vi "Read_Map.vi"(8 "error_in":errorcluster, 11 "Image In":T1) -> (0 "error out":errorcluster)   [LabVIEW 2020]
uses:
  <vilib>/vision/Image Controls.llb/IMAQ Image.ctl
  <vilib>/vision/NI_Vision_Development_Module.lvlib
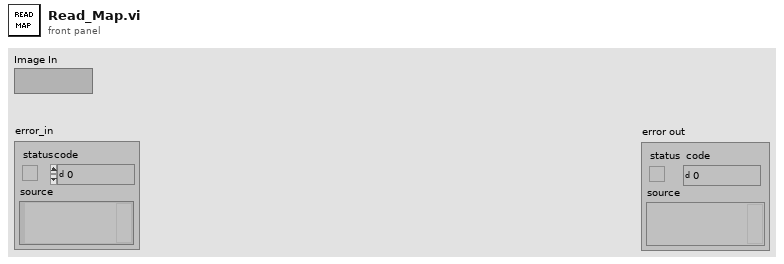
[diagram p1: front panel]
types:
  T1 = typedef "IMAQ Image.ctl" = refnum<image>
  T2 = typedef "Image_Cluster.ctl" = cluster{"Detector_info":cluster{"No. of detectors":dbl, "Detector_Array":string[][], "Detector_Array_Numeric":dbl[][]}, "Corner_info":cluster{"Corner_Array":dbl[][]}, "ROI":cluster{"Corners":cluster{"Global Rectangle":i32[], "Contours":cluster{"ID":enum32{"External", "Internal"}, "Type":u32, "Coordinates":i32[]}[]}[], "Detectors":cluster{"Global Rectangle":i32[], "Contours":cluster{"ID":enum32{"External", "Internal"}, "Type":u32, "Coordinates":i32[]}[]}[]}, "Shape_Detect":cluster{"Match_score":dbl, "Curve Parameters":T3, "Match Options":T4, "Circle Descriptor":cluster{"Min Radius":dbl, "Max Radius":dbl}}, "Path":cluster{"Config":path, "Map":path}, "Map":cluster{"X_resolution":i32, "Y_resolution":i32, "Image":T1}, "Conversion_factor":dbl}
  T3 = typedef "IMAQ Curve Parameters.ctl" = cluster{"Extraction Mode":u32, "Edge Threshold":i32, "Edge Filter Size":u32, "Min Length":i32, "Row Search Step Size":i32, "Col Search Step Size":i32, "Max Endpoint Gap":i32, "Closed":bool, "Subpixel":bool}
  T4 = typedef "ShapeDetectionMatchOptions.ctl" = cluster{"Rotation":bool, "Scale":bool, "Occlusion":bool, "Range Settings":T5[]}
  T5 = typedef "IMAQ Match Range Setting.ctl" = cluster{"Match Constraints":u32, "Min":dbl, "Max":dbl}
  T6 = cluster{"Global Rectangle":i32[], "Contours":cluster{"ID":enum32{"External", "Internal"}, "Type":u32, "Coordinates":i32[]}[]}[]
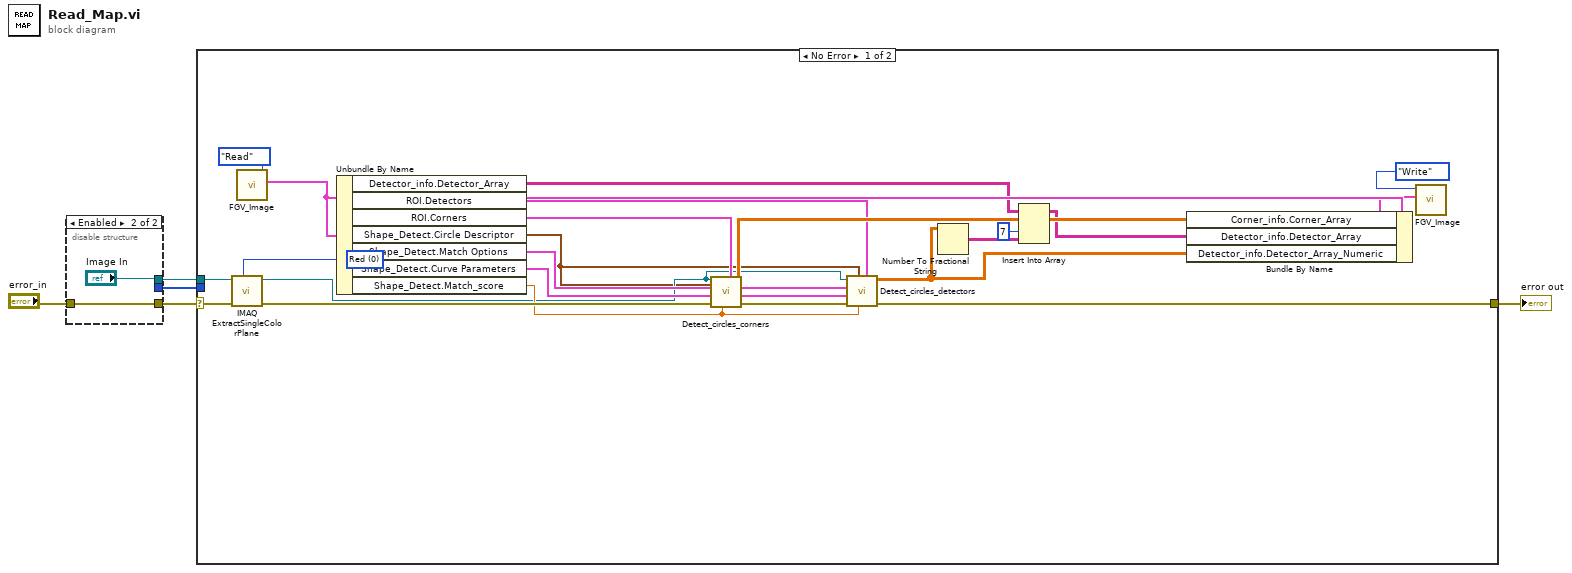
[diagram p0: block diagram]
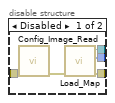
[diagram p2: hidden frame]
diagram:
  n1 = disable-structure shown="Enabled" {
    disable-tunnel: [w10 w12] -> w5
    disable-tunnel: [w9 "Image In"] -> w4
    disable-tunnel: [w8 _] -> w3
    disable-tunnel: "error_in" -> [w7 w12]
    frame Disabled {
      n2 = call "Config_Image_Read.vi"("error in (no error)"=w7) -> ("error out"=w6:errorcluster)  [unwired: 10 in]
      n3 = call "Load_Map.vi"("error in (no error)"=w6) -> ("error out"=w10:errorcluster, "image size"=w8:i32[], "Image Out"=w9:T1)  [unwired: 7 in]
    }
    frame Enabled {
    }
  }
  n4 = case shown="No Error" w5 {
    selector: w5 -> [w34 w36]
    tunnel: w4 -> [w35 _]
    tunnel: w3 -> [_ _]
    tunnel: [w24 w36] -> w2
    frame No Error {
      w26 = 0 items=["Red", "Green", "Blue", "Hue", "Saturation", "Luminance", "Value", "Intensity"] ("Color Plane")
      n5 = call "IMAQ ExtractSingleColorPlane"("Color Plane"=w26, "error in (no error)"=w34, "Image Src"=w35) -> ("error out"=w27:errorcluster, "Image Dst Out"=w20:T1)  [unwired: 1 in, 6 out]
      n6 = call "FGV_Image.vi"("Action"=enum16{"Read", "Write", ""}."Read") -> ("Image_Cluster_out"=w30:T2)  [unwired: 10 in]
      n7 = Unbundle By Name(w30) -> ("Detector_info.Detector_Array"=w16:string[][], "ROI.Detectors"=w18:T6, "ROI.Corners"=w32:T6, "Shape_Detect.Circle Descriptor"=w19:cluster{"Min Radius":dbl, "Max Radius":dbl}, "Shape_Detect.Match Options"=w21:T4, "Shape_Detect.Curve Parameters"=w22:T3, "Shape_Detect.Match_score"=w23:dbl)
      n8 = call "Detect_circles_corners.vi"("Corners"=w32, "Match_score"=w23, "Circle Descriptor"=w19, "error in (no error)"=w27, "Curve Parameters"=w22, "Match Options"=w21, "Refnum in"=w20) -> ("error out"=w25:errorcluster, "Array"=w28:sgl[][])  [unwired: 3 in]
      n9 = call "Detect_circles_detectors.vi"("Detectors"=w18, "Match_score"=w23, "Circle Descriptor"=w19, "error in (no error)"=w25, "Curve Parameters"=w22, "Match Options"=w21, "Refnum in"=w20) -> ("error out"=w24:errorcluster, "Array"=w17:sgl[][])  [unwired: 3 in]
      n10 = Number To Fractional String(number=w17) -> (F-format string=w15:string[][])  [unwired: 3 in]
      n11 = Insert Into Array(array=w16, index (col)=7 ("disabled index (col)"), new element=w15) -> (w14:string[][])  [unwired: 1 in]
      n12 = Bundle By Name(cluster=w30, "Corner_info.Corner_Array"=w28, "Detector_info.Detector_Array"=w14, "Detector_info.Detector_Array_Numeric"=w17) -> (w29:T2)
      n13 = call "FGV_Image.vi"("Image_Cluster_in"=w29, "Action"=enum16{"Read", "Write", ""}."Write") -> ()  [unwired: 9 in, 1 out]
    }
    frame Error {
    }
  }
  "error out" <- w2
